vi "from string.vi"(8 "error in":errorcluster, 9 "channel data":string, 10 "identifier":string, 11 "channel in":refnum<class "Modbus Module Channel.lvclass">) -> (0 "error out":errorcluster, 3 "channel out":refnum<class "Modbus Module Channel.lvclass">)   [LabVIEW 2014, in "Modbus Module Channel.lvclass"]
doc: "NI Tag Bus Module Framework 1.0.2.36\nNI Systems Engineering"
uses:
  Modbus Module Channel.lvclass
  <vilib>/NI/Tag Bus/tag/Data Type.ctl
  <vilib>/NI/Tag Bus Module Framework/channel/channel classification.ctl
  data bank type.ctl
  <vilib>/NI/Tag Bus/tag/tag descriptor.lvclass/tag descriptor.ctl
  <vilib>/NI/Tag Bus Module Framework/channel/TBM channel.lvclass/TBM channel.ctl
  Modbus Module Channel.lvclass/Modbus Module Channel.ctl
  <vilib>/NI/Tag Bus/tag/write tag name.vi
  <vilib>/NI/Tag Bus/tag/write raw default value.vi
  <vilib>/NI/Tag Bus/tag/write metadata.vi
  <vilib>/NI/Tag Bus/tag/write data type.vi
  <vilib>/NI/Tag Bus Module Framework/channel/Write channel classification.vi
  Write modbus type.vi
  Write starting address.vi
  Write subindex (bool).vi
  <vilib>/NI/Tag Bus/tag/tag descriptor.lvclass
  <vilib>/NI/Tag Bus Module Framework/channel/TBM channel.lvclass
  <vilib>/NI/Configuration Framework/serializable configuration/NISE_CEF_serializable configuration.lvclass
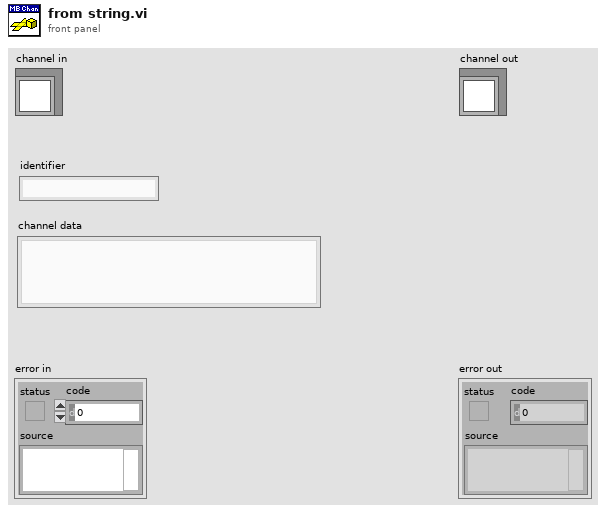
[diagram p1: front panel]
types:
  T1 = typedef "Modbus Module Channel.lvclass/data bank type.ctl" = enum16{"Coils", "Discrete Inputs", "Input Registers", "Holding Registers"}
  T2 = typedef "TBM channel.lvclass/channel classification.ctl" = enum16{"input data", "output data", "processing parameter", "processing result"}
  T3 = typedef "tag bus.lvlib/tag descriptor.lvclass/Data Type.ctl" = enum16{"Double", "Single", "I64", "I32", "I16", "I8", "U64", "U32", "U16", "U8", "Boolean", "String", "Array of Double", "Array of Single", "Array of I64", "Array of I32", "Array of I16", "Array of I8", "Array of U64", "Array of U32", "Array of U16", "Array of U8", "Array of Boolean", "Array of String"}
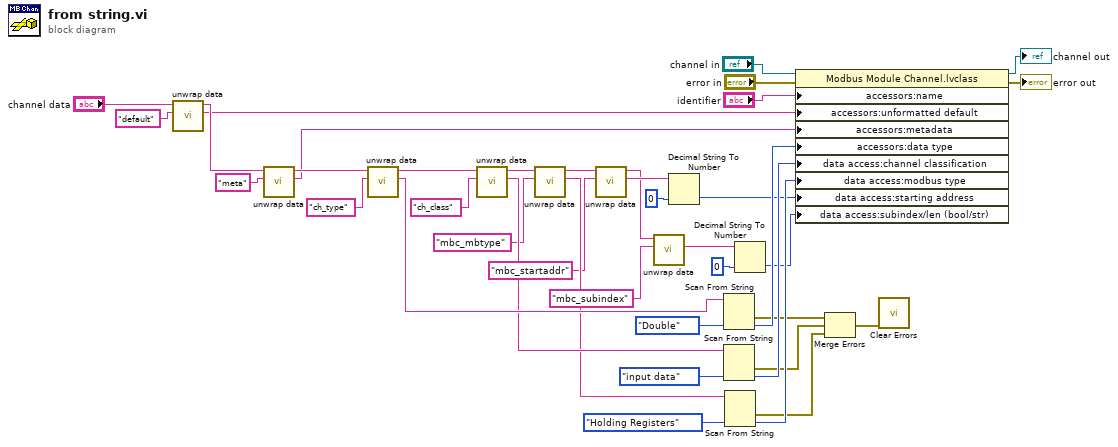
[diagram p0: block diagram]
diagram:
  n1 = call <vilib>:"unwrap data.vi"("identifier"="default", "data to unwrap"="channel data") -> ("unwrapped data"=w27:string, "remaining string"=w40:string)  [unwired: 8 in]
  n2 = call <vilib>:"unwrap data.vi"("identifier"="meta", "data to unwrap"=w40) -> ("unwrapped data"=w26:string, "remaining string"=w36:string)  [unwired: 8 in]
  n3 = call <vilib>:"unwrap data.vi"("identifier"="ch_type", "data to unwrap"=w36) -> ("unwrapped data"=w33:string, "remaining string"=w37:string)  [unwired: 8 in]
  n4 = call <vilib>:"unwrap data.vi"("identifier"="ch_class", "data to unwrap"=w37) -> ("unwrapped data"=w31:string, "remaining string"=w16:string)  [unwired: 8 in]
  n5 = call <vilib>:"unwrap data.vi"("identifier"="mbc_mbtype", "data to unwrap"=w16) -> ("unwrapped data"=w13:string, "remaining string"=w15:string)  [unwired: 8 in]
  n6 = call <vilib>:"unwrap data.vi"("identifier"="mbc_startaddr", "data to unwrap"=w15) -> ("unwrapped data"=w14:string, "remaining string"=w7:string)  [unwired: 8 in]
  n7 = call <vilib>:"unwrap data.vi"("identifier"="mbc_subindex", "data to unwrap"=w7) -> ("unwrapped data"=w9:string)  [unwired: 8 in, 1 out]
  n8 = Decimal String To Number(string=w14, default (0L)=u16 0 ("default (0 I32)")) -> (number=w18:u16)  [unwired: 1 in, 1 out]
  n9 = Scan From String(input string=w33, default 1=Data_Type."Double" ("data type")) -> (error out=w4:errorcluster, output 1=w25:T3)  [unwired: 3 in, 2 out]
  n10 = Scan From String(input string=w31, default 1=channel_classification."input data" ("channel classification")) -> (error out=w3:errorcluster, output 1=w24:T2)  [unwired: 3 in, 2 out]
  n11 = Scan From String(input string=w13, default 1=data_bank_type."Holding Registers" ("modbus type")) -> (error out=w2:errorcluster, output 1=w19:T1)  [unwired: 3 in, 2 out]
  n12 = Decimal String To Number(string=w9, default (0L)=0 ("default (0 I32)")) -> (number=w6:i32)  [unwired: 1 in, 1 out]
  n13 = property class="Modbus Module Channel.lvclass"(reference="channel in", error in="error in", "accessors:name"="identifier", "accessors:unformatted default"=w27, "accessors:metadata"=w26, "accessors:data type"=w25, "data access:channel classification"=w24, "data access:modbus type"=w19, "data access:starting address"=w18, "data access:subindex/len (bool/str)"=w6) -> (reference out=→"channel out":refnum<class "Modbus Module Channel.lvclass">, error out=→"error out":errorcluster)
  n14 = Merge Errors(w4, w3, w2) -> (w1:errorcluster)
  n15 = call <vilib>:"Clear Errors.vi"("error in (no error)"=w1) -> ()  [unwired: 5 in, 2 out]
